vi "DeleteAll.vi"(8 "error in (no error)":errorcluster) -> (0 "error out":errorcluster)   [LabVIEW 2014, in "Map Data.lvlib"]
doc: "Updates an existing contact or inserts a new contact into the address book data store. Use the ID of an existing contact to update, or an ID of 0 to insert. When inserting, the output cluster will contain the ID of the new contact."
uses:
  Map Data.lvlib
  MapCommand.ctl
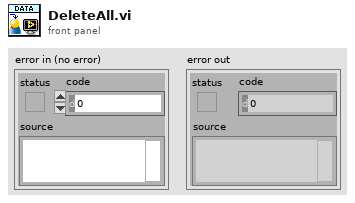
[diagram p1: front panel]
types:
  T1 = typedef "Map Data.lvlib/MapCommand.ctl" = enum16{"Load", "Update Cursor", "Save", "Get All Data", "Get Single Data", "Set Single Data", "Delete All", "Remove Single Data", "Set Favorite Status", "Is Data Modified", "Import Data"}
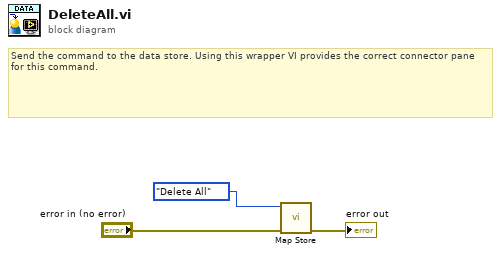
[diagram p0: block diagram]
diagram:
  # "Send the command to the data store. Using this wrapper VI provides the correct connector pane for this command."
  n1 = call "Map Store.vi"("error in (no error)"="error in (no error)", "Command"=MapCommand."Delete All") -> ("error out"=→"error out":errorcluster)  [unwired: 6 in, 3 out]
